vi "Compute Condition.vi"(0 "Joystick Guidance in":refnum<class "Joystick Guidance.lvclass">, 1 "X-Axis":dbl, 2 "Y-Axis":dbl, 3 "Z-Axis":dbl, 4 "Z-Axis Rotation":dbl, 5 "error in (no error)":errorcluster, 7 "Loop Nr":i32, 9 "First":bool) -> (14 "Joystick Guidance out":refnum<class "Joystick Guidance.lvclass">, 19 "error out":errorcluster)   [LabVIEW 2014, in "Guidance Library.lvlib" / "Joystick Guidance.lvclass"]
uses:
  Joystick Guidance.lvclass
  Joystick Guidance.lvclass/Joystick Guidance.ctl
  <vilib>/imath/engines/lvmath2/RunTimeEngine/Managers/WorkSpace/UID Generator.vi
  <vilib>/imath/engines/lvmath2/RunTimeEngine/RunTimeType/NIMS_RunTimeType_From StrictType (excl LVString).vi
  <instcachedir>/0/NIMS_RunTimeType_From StrictType (excl LVString)_15A5391EEA9C4AACB9955AC755B83D29.lvgen/NIMS_RunTimeType_From StrictType (excl LVString)_15A5391EEA9C4AACB9955AC755B83D29_008.vi
  <vilib>/imath/engines/lvmath2/RunTimeEngine/Struct/NIMS_StructSetField.vi
  <instcachedir>/0/NIMS_RunTimeType_From StrictType (excl LVString)_15A5391EEA9C4AACB9955AC755B83D29.lvgen/NIMS_RunTimeType_From StrictType (excl LVString)_15A5391EEA9C4AACB9955AC755B83D29_000.vi
  <vilib>/imath/engines/lvmath2/RunTimeEngine/RunTimeType/NIMS_RunTimeType_Set Source Original Bool.vi
  <vilib>/imath/engines/lvmath2/RunTimeEngine/LocalVariableDefStatement/MC_LocalVariableDefStatement_Display.vi
  <vilib>/imath/engines/lvmath2/RunTimeEngine/IndexReplace/NIMS V(R2)=S.vi
  <instcachedir>/0/NIMS V(R2)=S_913497CBBE4C412FA4D660FBDDEE588F.lvgen/NIMS V(R2)=S_913497CBBE4C412FA4D660FBDDEE588F_000.vi
  <vilib>/imathl/engines/lvmath/Functions/Error Handling/Create Error.vi
  <vilib>/imath/engines/lvmath2/RunTimeEngine/Struct/NIMS_StructGetField.vi
  <vilib>/imath/engines/lvmath2/RunTimeEngine/RunTimeType/NIMS_RunTimeType_To Numeric.vi
  <instcachedir>/0/NIMS_RunTimeType_To Numeric_CEDD3DBADEB64FB59CD8C53099B6B149.lvgen/NIMS_RunTimeType_To Numeric_CEDD3DBADEB64FB59CD8C53099B6B149_008.vi
  <vilib>/imath/engines/lvmath2/RunTimeEngine/IndexReplace/NIMS V(S)=S.vi
  <instcachedir>/0/NIMS V(S)=S_2D52C4EC15D8415E870AEE69FB516CCA.lvgen/NIMS V(S)=S_2D52C4EC15D8415E870AEE69FB516CCA_005.vi
  <vilib>/imath/engines/lvmath2/RunTimeEngine/IndexRead/NIMS V(S).vi
  <instcachedir>/0/NIMS V(S)_0488751826AF41519A22953C041130DC.lvgen/NIMS V(S)_0488751826AF41519A22953C041130DC_006.vi
  <vilib>/imath/engines/lvmath2/RunTimeEngine/ErrorHandling/NIMS_Create Error From Enums.vi
  <vilib>/imath/engines/lvmath2/RunTimeEngine/Managers/SymbolTable/Clear UID.vi
  <vilib>/imath/engines/lvmath2/RunTimeEngine/NodeEndStatement/NIMS_NodeEndStatement_Output.vi
  <instcachedir>/0/NIMS_NodeEndStatement_Output_53EC0D466D134D7ABD903AC30B43404B.lvgen/NIMS_NodeEndStatement_Output_53EC0D466D134D7ABD903AC30B43404B_015.vi
  <vilib>/imath/engines/lvmath2/RunTimeEngine/ErrorHandling/NIMS_Finalize Error.vi
  <vilib>/imath/engines/lvmath2/RunTimeEngine/Managers/SymbolTable/NIMS_WorkSpace.lvlib
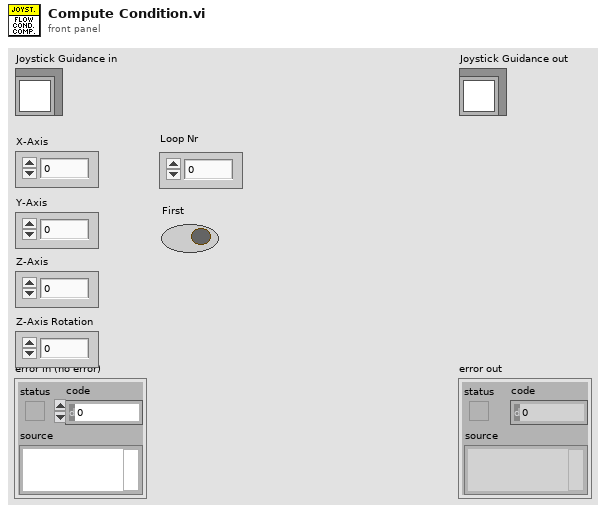
[diagram p1: front panel]
types:
  T1 = cluster{"X_Axis":bool, "Y_Axis":bool, "Z_Axis":bool, "Z_Axis_Rotation":bool}
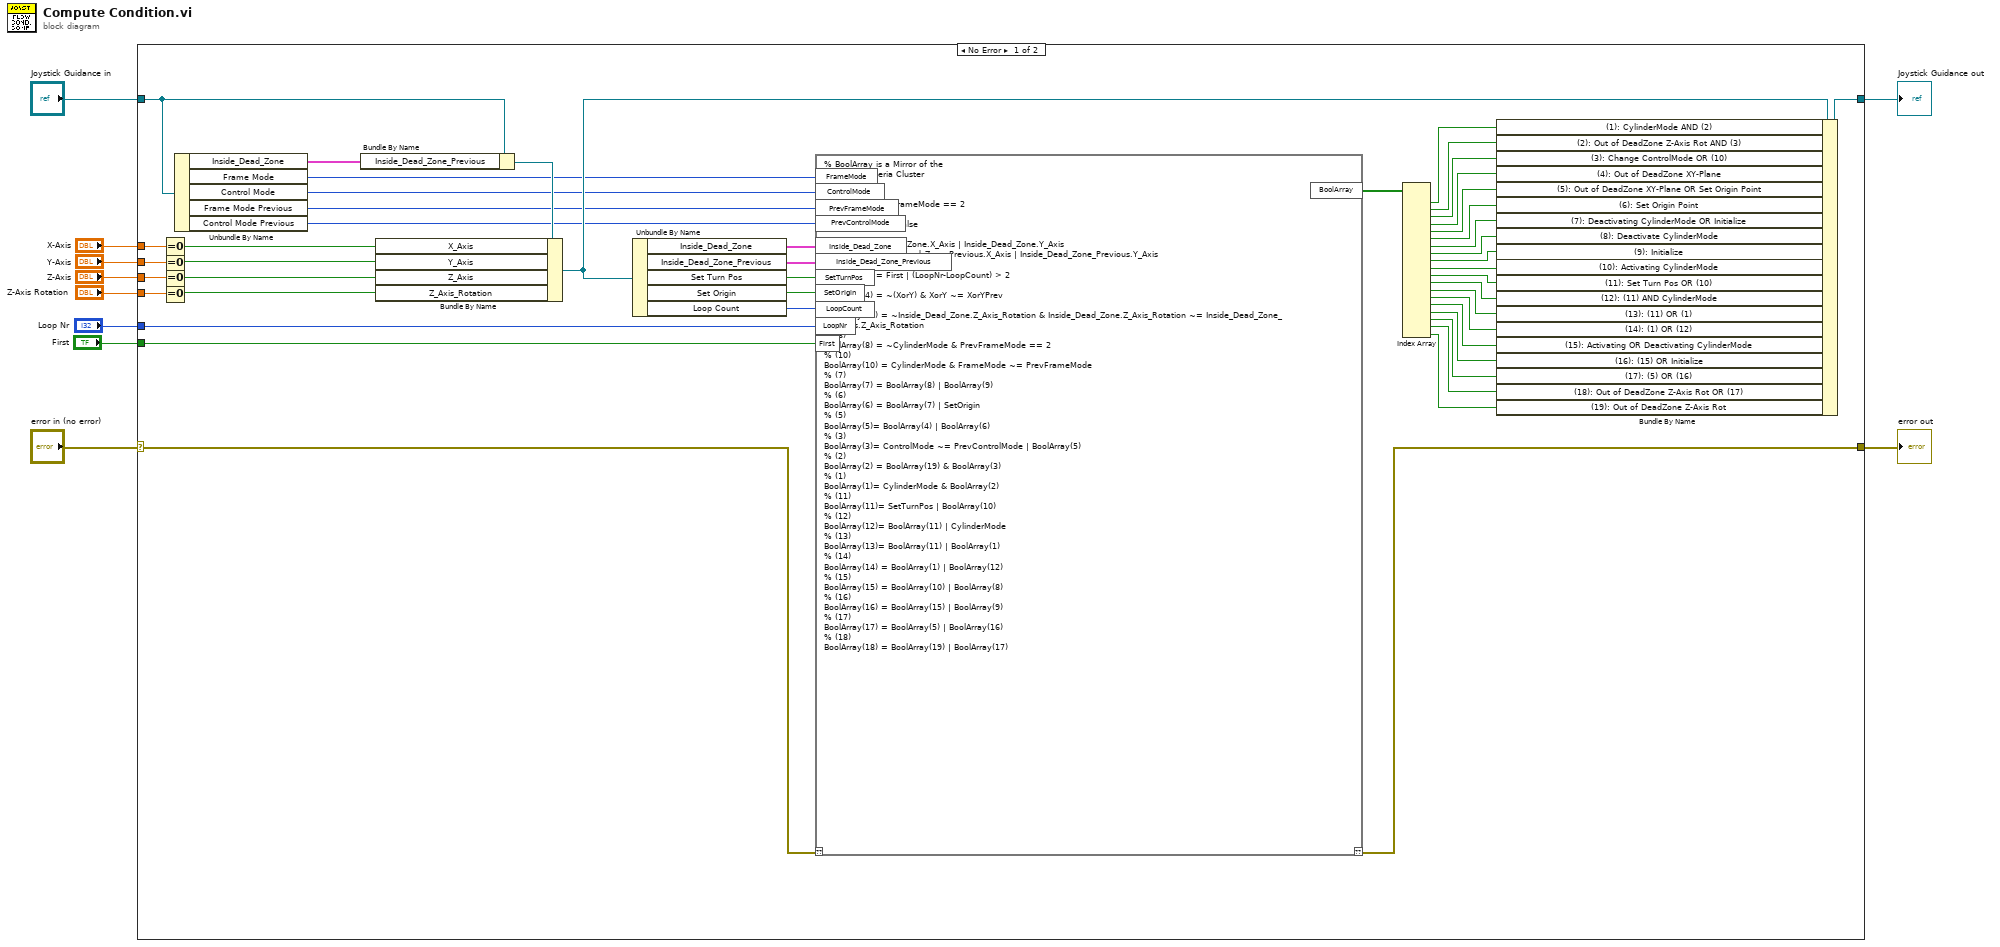
[diagram p0: block diagram]
diagram:
  n1 = case shown="No Error" "error in (no error)" {
    selector: "error in (no error)" -> [w16 w989]
    tunnel: [w15 w989] -> w9
    tunnel: [w48 w988] -> w7
    tunnel: "Joystick Guidance in" -> [w47 w988]
    tunnel: "X-Axis" -> [w56 _]
    tunnel: "Y-Axis" -> [w55 _]
    tunnel: "Z-Axis" -> [w54 _]
    tunnel: "Z-Axis Rotation" -> [w53 _]
    tunnel: "Loop Nr" -> [w14 _]
    tunnel: "First" -> [w11 _]
    frame No Error {
      n2 = Equal To 0?(x=w56) -> (x = 0?=w52:bool)
      n3 = Equal To 0?(x=w55) -> (x = 0?=w51:bool)
      n4 = Equal To 0?(x=w54) -> (x = 0?=w50:bool)
      n5 = Equal To 0?(x=w53) -> (x = 0?=w44:bool)
      n6 = Unbundle By Name(w47) -> ("Inside_Dead_Zone"=w46:T1, "Frame Mode"=w43:u16, "Control Mode"=w38:u16, "Frame Mode Previous"=w41:u16, "Control Mode Previous"=w42:u16)
      n7 = Bundle By Name(cluster=w47, "Inside_Dead_Zone_Previous"=w46) -> (w49:refnum<class "Joystick Guidance.lvclass">)
      n8 = Bundle By Name(cluster=w49, "X_Axis"=w52, "Y_Axis"=w51, "Z_Axis"=w50, "Z_Axis_Rotation"=w44) -> (w45:refnum<class "Joystick Guidance.lvclass">)
      n9 = Unbundle By Name(w45) -> ("Inside_Dead_Zone"=w40:T1, "Inside_Dead_Zone_Previous"=w39:T1, "Set Turn Pos"=w17:bool, "Set Origin"=w12:bool, "Loop Count"=w13:i32)
      n10 = mathscript code="% BoolArray is a Mirror of the \n%VI Flow Criteria Cluster\n\n% 1\nCylinderMode = FrameMode == 2\n\nBoolArray(1:19) = false\n\nXorY = Inside_Dead_Zone.X_Axis | Inside_Dead_Zone.Y_Axis\nXorYPrev = Inside_Dead_Zone_Previous.X_Axis | Inside_Dead_Zone_Previous.Y_Axis\n% (9)\nBoolArray(9) = First | (LoopNr-LoopCount) > 2\n% (4)\nBoolArray(4) = ~(XorY) & XorY ~= XorYPrev\n% (19)\nBoolArray(19) = ~Inside_Dead_Zone.Z_Axis_Rotation & Inside_Dead_Zone.Z_Axis_Rotation ~= Inside_Dead_Zone_Previous.Z_Axis_Rotation\n% (8)\nBoolArray(8) = ~CylinderMode & PrevFrameMode == 2\n% (10)\nBoolArray(10) = CylinderMode & FrameMode ~= PrevFrameMode\n% (7)\nBoolArray(7) = BoolArray(8) | BoolArray(9)\n% (6)\nBoolArray(6) = BoolArray(7) | SetOrigin\n% (5)\nBoolArray(5)= BoolArray(4) | BoolArray(6)\n% (3)\nBoolArray(3)= ControlMode ~= PrevControlMode | BoolArray(5)\n% (2)\nBoolArray(2) = BoolArray(19) & BoolArray(3)\n% (1)\nBoolArray(1)= CylinderMode & BoolArray(2)\n% (11)\nBoolArray(11)= SetTurnPos | BoolArray(10)\n% (12)\nBoolArray(12)= BoolArray(11) | CylinderMode\n% (13)\nBoolArray(13)= BoolArray(11) | BoolArray(1)\n% (14)\nBoolArray(14) = BoolArray(1) | BoolArray(12)\n% (15)\nBoolArray(15) = BoolArray(10) | BoolArray(8)\n% (16)\nBoolArray(16) = BoolArray(15) | BoolArray(9)\n% (17)\nBoolArray(17) = BoolArray(5) | BoolArray(16)\n% (18)\nBoolArray(18) = BoolArray(19) | BoolArray(17)"("??"=w16, "FrameMode"=w43, "ControlMode"=w38, "PrevFrameMode"=w41, "PrevControlMode"=w42, "Inside_Dead_Zone"=w40, "Inside_Dead_Zone_Previous"=w39, "LoopNr"=w14, "SetTurnPos"=w17, "SetOrigin"=w12, "LoopCount"=w13, "First"=w11) -> ("??"=w15:errorcluster, "BoolArray"=w37:bool[])
      n11 = Index Array(array=w37) -> (element #1=w36:bool, element #2=w35:bool, element #3=w34:bool, element #4=w33:bool, element #5=w32:bool, element #6=w31:bool, element #7=w30:bool, element #8=w29:bool, element #9=w28:bool, element #10=w27:bool, element #11=w26:bool, element #12=w25:bool, element #13=w24:bool, element #14=w23:bool, element #15=w22:bool, element #16=w21:bool, element #17=w20:bool, element #18=w19:bool, element #19=w18:bool)  [unwired: 19 in]
      n12 = Bundle By Name(cluster=w45, "(1): CylinderMode AND (2)"=w36, "(2): Out of DeadZone Z-Axis Rot AND (3)"=w35, "(3): Change ControlMode OR (10)"=w34, "(4): Out of DeadZone XY-Plane"=w33, "(5): Out of DeadZone XY-Plane OR Set Origin Point"=w32, "(6): Set Origin Point"=w31, "(7): Deactivating CylinderMode OR Initialize"=w30, "(8): Deactivate CylinderMode"=w29, "(9): Initialize"=w28, "(10): Activating CylinderMode"=w27, "(11): Set Turn Pos OR (10)"=w26, "(12): (11) AND CylinderMode"=w25, "(13): (11) OR (1)"=w24, "(14): (1) OR (12)"=w23, "(15): Activating OR Deactivating CylinderMode"=w22, "(16): (15) OR Initialize"=w21, "(17): (5) OR (16)"=w20, "(18): Out of DeadZone Z-Axis Rot OR (17)"=w19, "(19): Out of DeadZone Z-Axis Rot"=w18) -> (w48:refnum<class "Joystick Guidance.lvclass">)
    }
    frame Error {
    }
  }
  "error out" <- w9
  "Joystick Guidance out" <- w7
